vi "teste-motor-3-3.vi"() -> ()   [LabVIEW 2014]
doc: "André Romero - 2017\nandretec@ifsc.usp.br"
uses:
  C:/UserLabs/Andre/kinesis-lab14-32bits/kinesis-teste/Kinesis/Thorlabs.MotionControl.Controls.dll
  Kinesis/Thorlabs.MotionControl.Controls.dll
panel:
  out ".NET Refnum out 2":refnum<k24>
  out ".NET Refnum out":refnum<k24>
  out "Numeric 2":i32
  out "x-y":dbl
  out "GetPOS ABS 2":dbl=2.699072994402985
  out "GetPOS ABS 1":dbl=2.699072994402985
  in  "Ciclos":i32=100
  out "Numeric":i32
  out "GetPOS X":dbl=10.0 format="%#_6e"
  in  "GO Move":bool
  out "Motor 2":bool
  out "Motor 1":bool
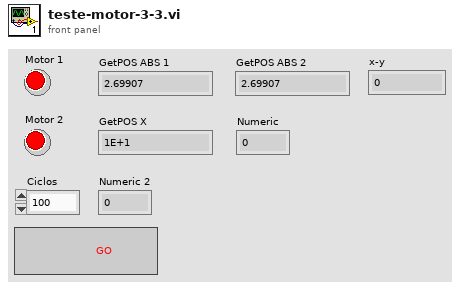
[diagram p1: front panel]
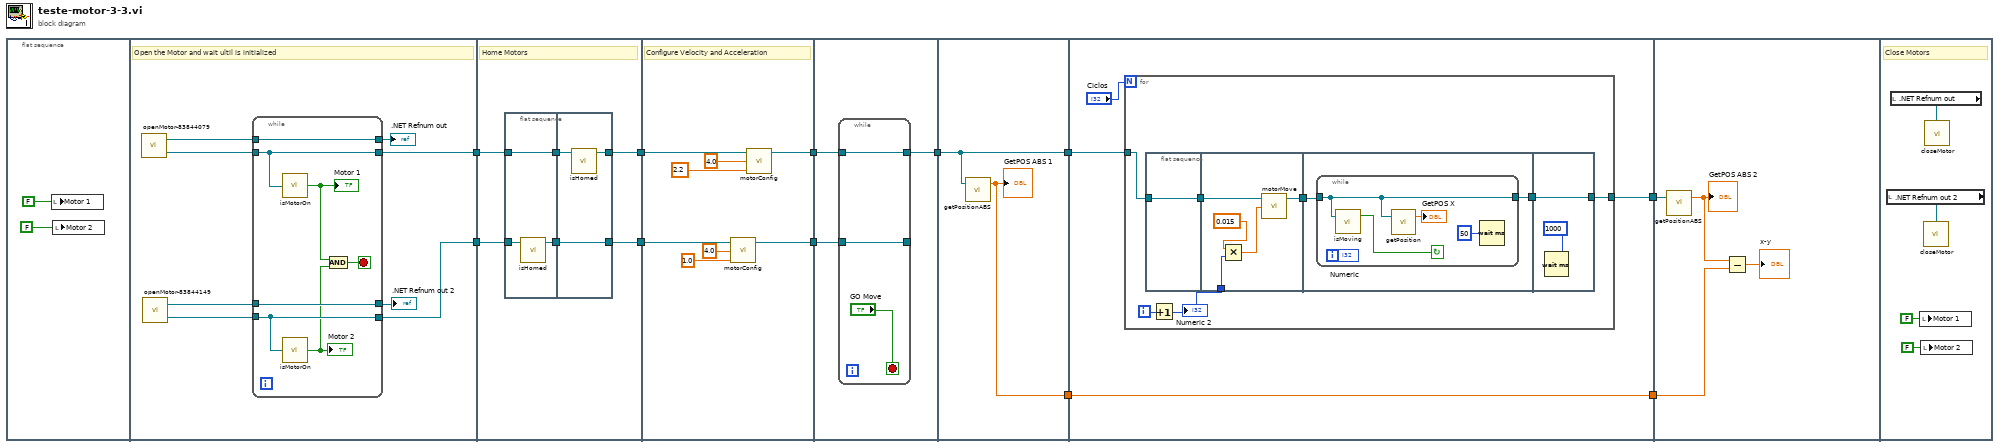
[diagram p0: block diagram]
diagram:
  n1 = flat-sequence {
    tunnel: [w19] -> w11
    tunnel: [w16] -> w10
    tunnel: w11 -> [w32]
    tunnel: [w33] -> w9
    tunnel: w10 -> [w34]
    tunnel: [w29] -> w7
    tunnel: w9 -> [w45]
    tunnel: [w41] -> w8
    tunnel: w7 -> [w48]
    tunnel: [w42] -> w6
    tunnel: w8 -> [w50]
    tunnel: w6 -> [w51]
    tunnel: [w49] -> w5
    tunnel: w5 -> [w56]
    tunnel: [w56] -> w4
    tunnel: [w55] -> w2
    tunnel: w4 -> [w59]
    tunnel: [w58] -> w3
    tunnel: w2 -> [w57]
    tunnel: [w57] -> w1
    tunnel: w3 -> [w86]
    tunnel: w1 -> [w83]
    frame #0 {
      n2 = local write "Motor 1"(FALSE ("isConnected")) -> ()
      n3 = local write "Motor 2"(FALSE ("isConnected 2")) -> ()
    }
    frame #1 {
      # "Open the Motor and wait ultil is initialized"
      n4 = call "openMotor-83844079.vi"() -> ("Device"=w20:refnum<k24>, ".NET Refnum out"=w21:refnum<k24>)  [unwired: 2 in]
      n5 = call "openMotor-83844149.vi"() -> ("Device"=w18:refnum<k24>, ".NET Refnum out"=w17:refnum<k24>)  [unwired: 2 in]
      n6 = while {
        tunnel: w21 -> [w28]
        tunnel: [w28] -> w15
        tunnel: w20 -> [w27]
        tunnel: [w27] -> w19
        tunnel: w18 -> [w25]
        tunnel: [w26] -> w14
        tunnel: w17 -> [w26]
        tunnel: [w25] -> w16
        stop <- w22 stop-if-true
        n7 = call "isMotorOn.vi"("Device"=w27) -> ("isConnected"=w23:bool)
        "Motor 1" <- w23
        n8 = call "isMotorOn.vi"("Device"=w25) -> ("isConnected"=w24:bool)
        "Motor 2" <- w24
        n9 = And(x=w23, y=w24) -> (x .and. y?=w22:bool)
      }
      ".NET Refnum out" <- w15
      ".NET Refnum out 2" <- w14
    }
    frame #2 {
      # "Home Motors"
      n10 = flat-sequence {
        tunnel: w34 -> [w37]
        tunnel: w32 -> [w35]
        tunnel: [w36] -> w31
        tunnel: [w35] -> w30
        tunnel: [w38] -> w29
        tunnel: [w40] -> w33
        tunnel: w31 -> [w40]
        tunnel: w30 -> [w39]
        frame #0 {
          n11 = call "isHomed.vi"("Device in"=w37) -> ("Device out"=w36:refnum<k24>)  [unwired: 4 in]
        }
        frame #1 {
          n12 = call "isHomed.vi"("Device in"=w39) -> ("Device out"=w38:refnum<k24>)  [unwired: 4 in]
        }
      }
    }
    frame #3 {
      # "Configure Velocity and Acceleration"
      n13 = call "motorConfig.vi"("Velocity"=1.0 ("MaxVelocity"), "Acceleration"=4.0, "Device in"=w45) -> ("Device out"=w41:refnum<k24>)  [unwired: 2 in]
      n14 = call "motorConfig.vi"("Velocity"=2.2 ("MaxVelocity"), "Acceleration"=4.0, "Device in"=w48) -> ("Device out"=w42:refnum<k24>)  [unwired: 2 in]
    }
    frame #4 {
      n15 = while {
        tunnel: [w53] -> w49
        tunnel: w51 -> [w53]
        tunnel: [w52] -> _
        tunnel: w50 -> [w52]
        stop <- "GO Move" stop-if-true
      }
    }
    frame #5 {
      n16 = call "getPositionABS.vi"("Device"=w56) -> ("GetPOS"=w55:dbl)  [unwired: 2 in]
      "GetPOS ABS 1" <- w55
    }
    frame #6 {
      n17 = for {
        N: "Ciclos" -> [_]
        tunnel: w59 -> [w66]
        tunnel: [w64] -> w58
        i -> [w63]
        n18 = flat-sequence {
          tunnel: [w68] -> w67
          tunnel: w66 -> [w68]
          tunnel: w67 -> [w73]
          tunnel: [w72] -> w65
          tunnel: w61 -> [w70]
          tunnel: w65 -> [w75]
          tunnel: [w74] -> w62
          tunnel: [w82] -> w64
          tunnel: w62 -> [w82]
          frame #0 {
          }
          frame #1 {
            n19 = Multiply(x=0.015 ("position"), y=w70) -> (x*y=w69:dbl)
            n20 = call "motorMove.vi"("position"=w69, "Device in"=w73) -> ("Device out"=w72:refnum<k24>)  [unwired: 3 in]
          }
          frame #2 {
            n21 = while {
              tunnel: w75 -> [w80]
              tunnel: [w80] -> w74
              i -> [w77]
              stop <- w79 continue-if-true
              n22 = call "isMoving.vi"("Device in"=w80) -> ("IsMoving"=w79:bool)  [unwired: 2 in]
              n23 = call "getPosition.vi"("Device"=w80) -> ("GetPOS"=→"GetPOS X":dbl)  [unwired: 2 in]
              n24 = Wait (ms)(milliseconds to wait=u32 50) -> ()  [unwired: 1 out]
              "Numeric" <- w77
            }
          }
          frame #3 {
            n25 = Wait (ms)(milliseconds to wait=u32 1000) -> ()  [unwired: 1 out]
          }
        }
        n26 = Increment(x=w63) -> (x+1=w61:i32)
        "Numeric 2" <- w61
      }
    }
    frame #7 {
      n27 = call "getPositionABS.vi"("Device"=w86) -> ("GetPOS"=w84:dbl)  [unwired: 2 in]
      "GetPOS ABS 2" <- w84
      n28 = Subtract(x=w84, y=w83) -> (x-y=→"x-y":dbl)
    }
    frame #8 {
      # "Close Motors"
      n29 = local read ".NET Refnum out 2"() -> (w87:refnum<k24>)
      n30 = local read ".NET Refnum out"() -> (w88:refnum<k24>)
      n31 = local write "Motor 1"(FALSE ("Motor 1")) -> ()
      n32 = local write "Motor 2"(FALSE ("Motor 2")) -> ()
      n33 = call "closeMotor.vi"(".NET Refnum in"=w87) -> ()  [unwired: 2 in]
      n34 = call "closeMotor.vi"(".NET Refnum in"=w88) -> ()  [unwired: 2 in]
    }
  }
